vi "Probe.vi"(8 "error in (no error)":errorcluster caption="entrée d'erreur (pas d'erreur)", 11 "Message":string) -> (0 "error out":errorcluster caption="sortie d'erreur")   [LabVIEW 2020, in "Library Test.lvlib" / "Test (Default).lvclass"]
uses:
  Test (Default).lvclass
  Core/Actors/Actor_Log/Actor_Log/Actor_Log Messages/Log Msg/Log Msg.lvclass/Log Msg.ctl
  <vilib>/ActorFramework/Message Enqueuer/Message Enqueuer.lvclass/Message Enqueuer.ctl
  <vilib>/ActorFramework/Message Enqueuer/Enqueue.vi
  Core/Actors/Actor_Log/Actor_Log/Actor_Log Messages/Log Msg/Log Msg.lvclass
  C:/Program Files (x86)/National Instruments/LabVIEW 2020/vi.lib/ActorFramework/Message/Message.lvclass
  <vilib>/ActorFramework/Message Priority Queue/Priority Enqueue.vi
  Commun VI/Library Commun.lvlib
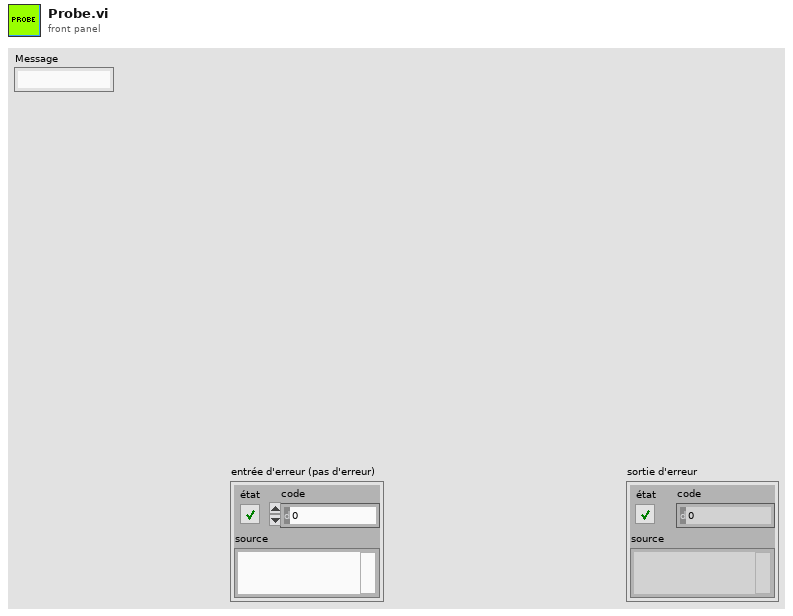
[diagram p1: front panel]
types:
  T1 = enum16{"Init", "Add Actor", "Delete Actor", "Get Actor Queue", "Get Log Actor Queue", "List all actors"}
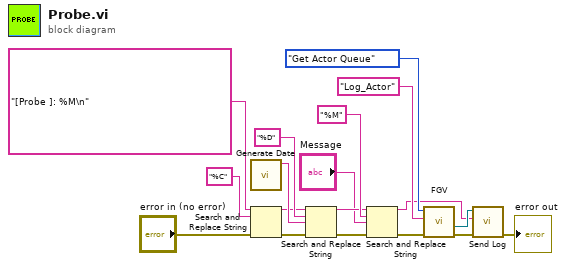
[diagram p0: block diagram]
diagram:
  n1 = call "Generate Date.vi"() -> ("chaîne de date/heure"=w10:string)  [unwired: 11 in]
  n2 = Search and Replace String(input string="[Probe ]: %M\n", search string="%C", error in="error in (no error)") -> (result string=w1:string, error out=w9:errorcluster)  [unwired: 5 in, 2 out]
  n3 = Search and Replace String(input string=w1, search string="%D", replace string=w10, error in=w9) -> (result string=w4:string, error out=w5:errorcluster)  [unwired: 4 in, 2 out]
  n4 = Search and Replace String(input string=w4, search string="%M", replace string="Message", error in=w5) -> (result string=w2:string, error out=w8:errorcluster)  [unwired: 4 in, 2 out]
  n5 = call "FGV.vi"("error in (no error)"=w8, "Actor name"="Log_Actor", "Action"=T1."Get Actor Queue") -> ("error out"=w15:errorcluster, "Actor's Queue Out"=w16:refnum<class "Message Enqueuer.lvclass">)  [unwired: 6 in, 1 out]
  n6 = call "Send Log.vi"("error in (no error)"=w15, "String to add"=w2, "Message Enqueuer"=w16) -> ("error out"=→"error out":errorcluster)  [unwired: 7 in, 1 out]
